vi "Redraw.vi"(8 "error in (no error)":errorcluster, 11 "HistorianCharting in":refnum<class "HistorianCharting.lvclass">) -> (0 "error out":errorcluster, 3 "HistorianCharting out":refnum<class "HistorianCharting.lvclass">)   [LabVIEW 2020, in "VolatusGUIElements.lvlib" / "HistorianCharting.lvclass"]
uses:
  HistorianCharting.lvclass
  HistorianCharting.lvclass/HistorianCharting.ctl
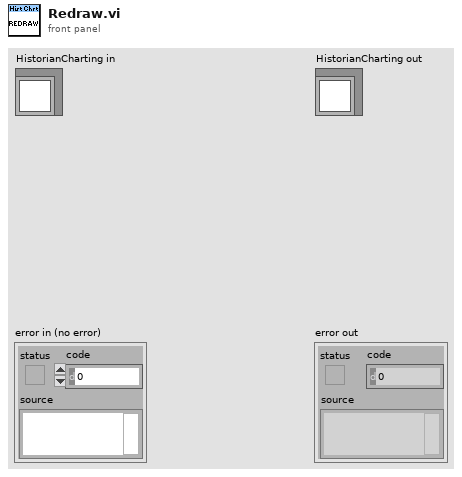
[diagram p1: front panel]
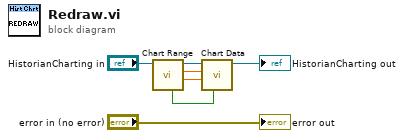
[diagram p0: block diagram]
diagram:
  n1 = call "Chart Range.vi"("HistorianCharting in"="HistorianCharting in") -> ("End"=w2:dbl, "Start"=w3:dbl, "HistorianCharting out"=w5:refnum<class "HistorianCharting.lvclass">, "Set Time"=w1:bool)  [unwired: 6 in, 1 out]
  n2 = call "Chart Data.vi"("Set Time"=w1, "End"=w2, "Start"=w3, "HistorianCharting in"=w5) -> ("HistorianCharting out"=→"HistorianCharting out":refnum<class "HistorianCharting.lvclass">)  [unwired: 6 in, 1 out]
  "error out" <- "error in (no error)"
